vi "Is Nominal State.vi"(11 "Base Queue in":refnum<class "Base Queue.lvclass">) -> (2 "Is Nominal State?":bool)   [LabVIEW 2021, in "jettl.lvlib" / "Base Queue.lvlib" / "Base Queue.lvclass"]
uses:
  Base Queue.lvclass
  State/Nominal State/Nominal State.lvclass
  C:/git/jettl/jettl/jettl/Base Queue/State/State/State.lvclass
  Base Queue.lvclass/Base Queue.ctl
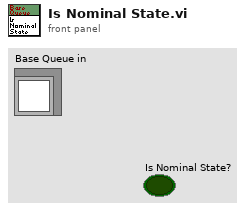
[diagram p1: front panel]
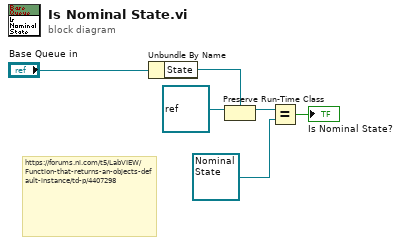
[diagram p0: block diagram]
diagram:
  # "https://forums.ni.com/t5/LabVIEW/Function-that-returns-an-objects-default-instance/td-p/4407298"
  n1 = Unbundle By Name("Base Queue in") -> ("State"=w5:refnum<class "State.lvclass">)
  n2 = Preserve Run-Time Class(object in=refnum<class> refnum ("LabVIEW Object"), 2:w5) -> (object out=w3:refnum<class "State.lvclass">)  [unwired: 1 in, 1 out]
  n3 = Equal?(x=w3, y=refnum<class "Nominal State.lvclass"> refnum ("jettl.lvlib:Base Queue.lvlib:State.lvlib:Nominal State.lvclass")) -> (x = y?=→"Is Nominal State?":bool)
